vi "evo irimager set shutter mode.vi"(11 "mode":i32) -> (3 "function return":i32)   [LabVIEW 2017, in "libirimager_direct_binding.lvlib"]
doc: "DIRECT_API int evo_irimager_set_shutter_mode(int mode);"
uses:
  libirimager_direct_binding.lvlib
  labview/libirimager.dll
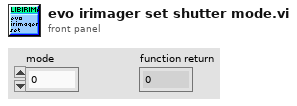
[diagram p1: front panel]
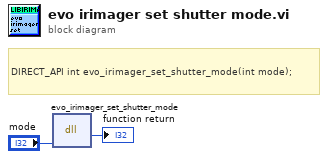
[diagram p0: block diagram]
diagram:
  # "DIRECT_API int evo_irimager_set_shutter_mode(int mode);"
  n1 = dll-call lib="C:/Users/HelmutEngelhardt/Documents/labview/libirimager.dll" fn="evo_irimager_set_shutter_mode"("mode"="mode") -> ("Rückgabetyp"=→"function return":i32)  [unwired: 4 in, 2 out]
